vi "Save Date.vi"(9 "Save Data":string[][](array[string]), 11 "布尔":bool) -> (1 "Save Data Out":string[][](array[string]))   [LabVIEW 2019]
panel:
  out "Save":string[][](array[string])
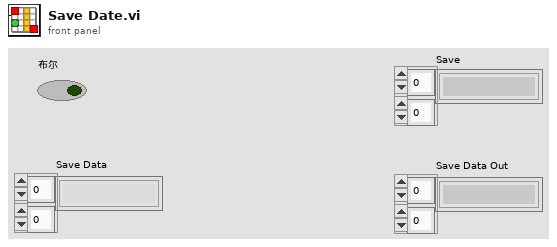
[diagram p1: front panel]
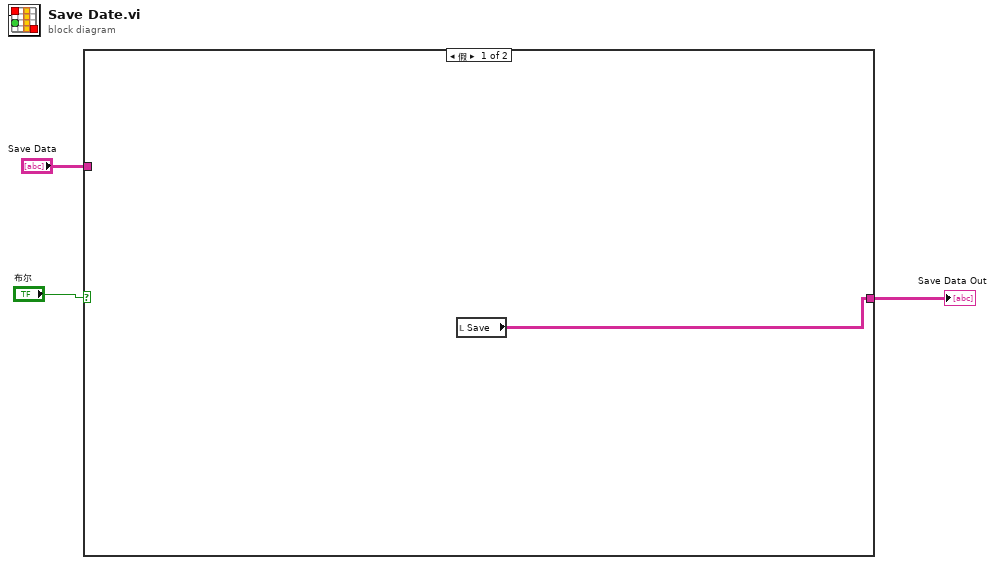
[diagram p0: block diagram]
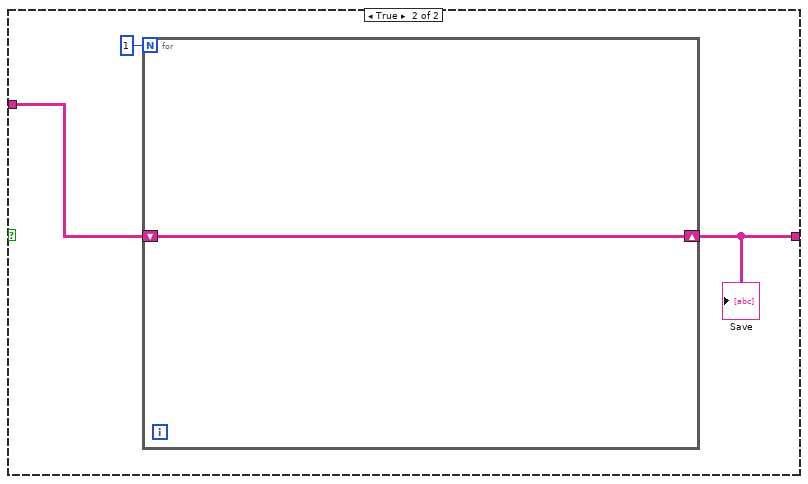
[diagram p2: hidden frame]
diagram:
  n1 = case shown="假" "布尔" {
    tunnel: "Save Data" -> [_ w6]
    tunnel: [w4 w5] -> w1
    frame False {
      n2 = local read "Save"() -> (w4:string[][])
    }
    frame True {
      n3 = for {
        N: 1 -> [_]
        shift-right: [w8] -> w5
        shift-left: w6 -> [w8]
      }
      "Save" <- w5
    }
  }
  "Save Data Out" <- w1
